vi "Measurement Logic.vi"() -> ()   [LabVIEW 2021, in "Crosstalk_Class D Amplifier.lvlib"]
uses:
  Crosstalk_Class D Amplifier.lvlib
  Measurement Configuration.ctl
  shared/controls/digital audio protocol/data justification.ctl
  shared/controls/digital audio protocol/endianness.ctl
  shared/controls/digital audio protocol/digital edge.ctl
  shared/controls/digital audio protocol/logic level.ctl
  shared/controls/output mode.ctl
  shared/controls/lowpass filter.ctl
  shared/controls/highpass filter.ctl
  Measurement Results.ctl
  <vilib>/MeasurementLink/MeasurementLink Measurement Server/Classes/MeasurementContext/MeasurementContext.lvclass
  <vilib>/PDM Acquisition Toolkit/shared/controls/clock mode.ctl
  <vilib>/PDM Acquisition Toolkit/shared/controls/PCM Frame Sync Control.ctl
  <vilib>/PDM Acquisition Toolkit/shared/controls/Digital Edge.ctl
  <vilib>/PDM Acquisition Toolkit/shared/controls/PCM Data Format Configuration.ctl
  <vilib>/PDM Acquisition Toolkit/shared/controls/PCM Bit Endianness.ctl
  <vilib>/PDM Acquisition Toolkit/shared/controls/PCM Data Justification.ctl
  shared/controls/audio filter settings.ctl
  shared/controls/weighting filter.ctl
  <vilib>/DAQmx/read.llb/DAQmx Read (Analog 1D Wfm NChan NSamp).vi
  <vilib>/addons/_NISVFA/_Shared subVIs/Common/SVL Set dB Reference (N Ch - 1 Ref).vi
  <vilib>/addons/_NISVFA/_Spectrum Processing/SVFA Unit Conversion (Complex) (1 Ch).vi
  <vilib>/addons/_NISVFA/_Shared subVIs/Common/SVL Set dB Reference (1 Ch).vi
  <vilib>/addons/_NISVFA/_Shared subVIs/Common/svc_Log View for Spectrum (1Ch).vi
  <vilib>/addons/_NISVFA/_Spectrum Processing/SVFA Unit Conversion (1 Ch).vi
  <vilib>/addons/_NISVFA/_Shared subVIs/Common/svc_Complex Datatype Defaults.vi
  <vilib>/addons/_NISVFA/_Shared subVIs/Common/SVL Set dB Reference (variant).vi
  <vilib>/addons/_NISVFA/_Shared subVIs/Common/svc_Unwrap Phase.vi
  <vilib>/addons/_NISVFA/_Shared subVIs/Common/svc_Convert Spectrum Array to dB.vi
  <vilib>/addons/_NISVFA/_Shared subVIs/Common/svc_Spectrum Units.vi
  <vilib>/addons/_NISVFA/_Spectrum Processing/subVIs/svfa_Conversion Utility (spectrum info).vi
  <vilib>/addons/_NISVFA/_Shared subVIs/Common/svc_Format Value (DBL).vi
  <vilib>/addons/_NISVFA/_Shared subVIs/Common/svc_Get Weighting Enum and Labels.vi
  <vilib>/addons/_NISVFA/_Shared subVIs/Common/svc_Engineering Units to Unit Label.vi
  <vilib>/addons/_NISVFA/_Shared subVIs/Common/svc_Surround NonAlpha String with Parentheses.vi
  <vilib>/dlg_ctls.llb/Space Constant.vi
  <vilib>/addons/_NISVFA/_Spectrum Processing/subVIs/svfa_Peak to RMS to Peak2Peak.vi
  <vilib>/addons/_NISVFA/_Spectrum Processing/subVIs/svfa_Mag to Mag2.vi
  <vilib>/addons/_NISVFA/_Spectrum Processing/subVIs/svfa_Linear to dB.vi
  <vilib>/addons/_NISVFA/_Spectrum Processing/subVIs/svfa_dBrefA to dBrefB.vi
  <vilib>/addons/_NISVFA/_Spectrum Processing/subVIs/svfa_Spectrum to Spectral Density.vi
  <vilib>/addons/_NISVFA/_Shared subVIs/Common/svc_Unit Label Lexical Class.vi
  <vilib>/addons/_NISVFA/_Shared subVIs/Common/svc_Window Parameters.vi
  <vilib>/PDM Acquisition Toolkit/host/API/Public/Function Generator/Configure Custom Signal (N Ch) - PCM Output Task.vi
  <vilib>/DAQmx/create/channels.llb/DAQmx Create Channel (AI-Voltage-Basic).vi
  <vilib>/DAQmx/configure/timing.llb/DAQmx Timing (Sample Clock).vi
  <vilib>/DAQmx/miscellaneous.llb/DAQmx Fill In Error Info.vi
  <vilib>/Waveform/WDTOps.llb/WDT Get Waveform Subset DBL.vi
  <vilib>/addons/_NISVFA/_Shared subVIs/Common/svc_Caller VI Returned in Error Source.vi
  <vilib>/addons/Sound and Vibration/svt_Single Tone Measurements/SVT Crosstalk (Time).vi
  <vilib>/Analysis/4window.llb/window parameters.vi
  <vilib>/Analysis/4window.llb/Window Properties.vi
  <vilib>/Analysis/4window.llb/Window Properties by Name.vi
  <vilib>/PDM Acquisition Toolkit/shared/PDM Shared.lvlib
  <vilib>/PDM Acquisition Toolkit/host/API/PDM Acquisition Toolkit.lvlib
  <vilib>/addons/Sound and Vibration/svt_Single Tone Measurements/SoundVib_SingleTone.lvlib
panel:
  out "crosstalk":dbl=-96.02835709393884 format="%.2f"
  out "Spectrum":cluster{"x0":dbl, "dx":dbl, "magnitude":dbl[]}[](graph)=[{"x0"=0.0, "dx"=10.00000000139779, "magnitude"=[-102.50662414333134, -98.42652990737129, -104.36739546360309, -114.71774418702175, -130.36950761428557, -151.23179944533624, -152.21861985637932, -146.68742010394863, -149.2705486874169, -158.8294889407479, -160.38776152909975, -149.09872862612403, -145.52257764827635, -146.94377835759036, -151.8503529216404, -149.495187799045, -146.71000188943978, -146.69467169532174, -147.12415322287058, -146.48101024151816, -146.11259440489056, -146.44367304019693, -147.16083048011208, -148.24952674145092, -150.7676188196385, -154.27917637865204, -150.59384849249707, -148.98529072383565, -151.80720194111765, -155.58360918997693, -151.8641272955873, -149.48762329108004, -149.21639953625385, -151.57158440849594, -157.76903119960159, -153.55378069412103, -151.44318082938975, -148.28996695923874, -144.44122146588828, -143.35252367233983, -144.67504951998674, -148.79447192432244, -162.68305251758406, -155.9956623734257, -153.88465520414786, -153.86437747010777, -148.21400992111495, -143.7975301951548, -141.60763781007233, -141.11798493153222, -141.7657625033544, -143.3439946619613, -147.27626397312403, -153.9129306331063, -150.10843385304614, -150.8646772606705, -157.21868893436113, -153.32467973484376, -148.2886012013035, -145.97763528730337, -145.02294775535685, -145.95380075725188, -148.52742611082346, -150.26860428681573, -149.80402808731668, -149.15784362193327, -148.88729473328095, -147.6410694225479, -146.1024386899084, -144.04164734740414, -141.8096017401985, -141.89909839162925, -144.33041994087705, -147.03168187155697, -149.8848916012044, -157.242108057668, -163.7020765469617, -154.84916895378942, -149.35365799485976, -149.84724642155038, -166.16154969079048, -150.02372164994102, -144.4812771299088, -143.00962426465077, -145.06223612725626, -150.044365326583, -145.22102393138212, -143.9047030742633, -147.6498522760554, -148.24512347909143, -144.57573215941838, -144.70421020795382, -149.3992307646427, -157.15858661145447, -149.53376442882706, -145.3500882194989, -130.51626677502895, -115.35893596609503, -104.94632092121802, -98.949745178228, -96.98127597071934, -98.91764337842676, -104.89188220482681, -115.35756716290187, -131.32460144183233, -146.02564661193153, -146.64746502318445, -146.20546432744308, -146.06344187627312, -146.71885957609217, -147.79386540056154, -148.3129984329201, -150.07404032747172, -151.01606867264618, -148.53275640333467, -148.87942637036383, -154.84736140480553, -163.03493024930194, -155.9886526254461, -152.9771504364054, -151.23934598346432, -152.1177287204616, -156.0415527622356, -155.79464630187738, -153.37427864278084, -158.35633010893818, -160.4917326183105, -152.35724216472744, -150.4085235923613, -149.8464780305325, -150.0858277076875, -152.5365543882359, -162.90001265859559, -154.99187315427372, -149.68230609250867, -149.6624222051648, -152.52015170412253, -158.53256622609155, -157.0591968458093, -151.9582556061719, -151.67400414787312, -153.67246366723705, -153.1115685027894, -148.62047969080592, -144.6077065989328, -143.19296640779524, -144.480175755617, -147.26987733162733, -148.8892501068937, -148.0514091905835, -147.536282157801, -148.14352395217057, -147.7677986743226, -146.105745543478, -145.90665814762045, -149.0691401536877, -156.57421189502384, -164.72882020791783, -159.6130972077308, -156.623446560449, -168.85104749052408, -150.1954388285173, -146.74490253016342, -146.42710082184223, -146.06109903695113, -145.11661710541068, -144.87553776047872, -144.76308854188835, -143.36594721535567, -141.29005284167016, -139.77326961768037, -139.65307685067194, -141.68570199128544, -146.42344929092278, -153.22082520634922, -157.77018729369573, -163.00672947759253, -155.66402624536914, -151.72600006433075, -151.90729513417844, -154.055798824148, -153.4554584753518, -149.91810848168632, -146.58444477553613, -144.63227084249445, -143.10913319168768, -142.44048469202568, -144.03441960908424, -150.1025256903153, -170.5464622355483, -160.5458487789234, -148.6474653914609, -142.26330840446758, -140.24130009354744, -141.15484410150341, -144.45679526342136, -151.16119262924147, -151.27648900881798, -142.80993347375116, -138.45182736457332, -137.28603898597132, -139.60807023724797, -145.8636544858835, -151.97115320990244, -151.04114645463892, -150.24123918473293, -149.6371510881664, -150.28927070808865, -150.77161085232433, -149.479675124508, -149.16415541371822, -148.33483632282497, -149.71946210000516, -165.2254495823216, -149.2903130550451, -145.09890222425162, -145.13108280185085, -144.55049294104808, -143.64986368181266, -143.8513304492729, -145.2452116463332, -148.08438161552965, -153.74551065668277, -150.97295897851075, -145.56111974259778, -144.2683578235665, -145.4377665440953, -148.485299942523, -150.606088512832, -149.99901231630875, -153.50105219162285, -157.23107319433217, -152.20302275714664, -155.10568917925568, -182.21878042594437, -155.79850642940846, -149.47657549067756, -146.03673660068378, -144.71418632430388, -144.64436135224898, -145.14852658463394, -146.49628233453257, -150.12506361661227, -159.39136861280997, -162.91970926440146, -163.2211796732435, -167.41114333754035, -159.92861809688566, -156.95423609482174, -150.13886796894343, -146.272968974304, -144.97270598274608, -145.71163317248636, -148.36936121203755, -151.52392886602624, -151.81294816394396, -148.4389448694476, -145.347254503234, -145.0137941154527, -146.21656114414765, -145.71446644721158, -144.26784782916442, -144.8517696110422, -149.3311559719114, -157.19623409642165, -153.14838913323788, -149.80264318689342, -149.51499154993155, -150.0562395375804, -150.46532838788946, -151.81512130027212, -152.08492889376294, -152.27886346828404, -152.96971224616814, -146.00946808785085, -142.63380182350278, -142.67257094910715, -144.48588408268375, -146.4574125986869, -146.8639541246159, -144.39989729111542, -142.6384852492207, -143.3405308391282, -146.01449041545808, -147.77110553826077, -146.78677258658166, -147.80286353597137, -152.5589981112538, -156.17665827599075, -153.973050299784, -154.463102201682, -157.43991958882845, -172.46200114292324, -154.9055892894335, -150.2440233565258, -148.90848142218192, -148.3678538030235, -144.37651973237894, -137.47177539760602, -132.94796185556405, -131.54941025908641, -133.09421788289777, -136.8607463694835, -140.9941498406433, -143.32980767027848, -142.84243382400552, -141.41290900729877, -141.9150734924524, -145.56876843523418, -152.59815574779995, -156.7145964730788, -153.53837597530674, -148.95303591584755, -146.66230348220537, -147.39801912671663, -152.81957024991863, -161.4774498516955, -164.16791044396444, -157.66737544153668, -149.95484667711608, -147.75064574787046, -147.6282926679159, -149.81435262545037, -157.1769895252467, -151.78442822013145, -146.9995200796308, -146.03971538945834, -147.77640124911764, -153.9215633435758, -152.60188744077465, -147.37187720270674, -148.43177928716185, -154.65248382464895, -153.95149291837828, -150.9825556620198, -152.29977978280488, -155.2390354869051, -149.08148104181603, -146.19449053515595, -145.4584987818286, -144.2566970344048, -142.8851826872422, -142.6395736808178, -143.48112329223648, -145.93250198901367, -146.55445027776247, -142.28911808864905, -141.0438316750318, -142.4606533936622, -142.9611355916092, -141.74906552128527, -141.17083672844248, -140.77562836032112, -140.4251709224202, -141.5784061337755, -145.27525608539767, -150.2568137811816, -151.97456113128104, -154.10586925167826, -149.4941602885088, -145.10021934337752, -144.95448872098984, -147.22959951845755, -148.5519093591704, -147.42151523913248, -146.31152370731377, -146.39765371113307, -148.1317610180549, -150.04644464092766, -149.14755515841532, -147.6734828207496, -147.41795159911305, -149.2077277894993, -153.87907767546167, -157.45178914332806, -156.68647377396408, -150.2656499600685, -145.0865782383265, -143.7527692106753, -145.415690876855, -149.4501875710815, -158.52042346703536, -157.8361480689608, -153.4137340474177, -157.30706432079694, -156.4141011095387, -151.83212675449715, -148.7923245236713, -146.32578579596012, -145.4762086973766, -147.26253749848811, -150.45310485787675, -150.6472259696284, -148.4730437307641, -147.85107501340758, -153.67423252222903, -154.10414907771943, -143.32770328199229, -138.0381077328083, -134.4834285265295, -133.5847497838884, -136.2414630969185, -142.09828818205534, -145.92943621139213, -145.24799642531607, -143.78887250522922, -144.08573780081082, -146.43011870617693, -147.15783195784863, -145.92004215266292, -145.68872987445536, -146.164833535183, -146.8753573776017, -147.82392725779468, -149.9187907131617, -155.00485040457747, -174.42491441876496, -155.66154280189093, -148.86628234318596, -145.19322816565062, -143.58136195052955, -144.13634952775777, -146.80034879832203, -149.61413931819257, -148.8639340265086, -146.55103578130888, -146.39749614389314, -149.93126167479267, -150.81086141741253, -146.58075107437048, -143.88919306899965, -142.58041660603087, -142.57992649086592, -143.60532930766522, -146.19675809957423, -152.03286235362984, -151.87476831617087, -148.67005434293947, -146.69500807908705, -144.84575426749163, -144.6292522850046, -146.29427139187112, -149.17942524652585, -152.527120738668, -155.49871242883344, -155.20088215079033, -151.4744693585207, -148.01318050378268, -147.16447927264923, -148.17440278636408, -151.2358775189423, -164.24094842320358, -153.54883070626144, -147.11115687456774, -143.18347079178054, -141.40634376329825, -142.0606833931419, -145.9862099123088, -157.70364335248402, -154.7432383392768, -151.14179490076916, -152.74577633516049, -153.8210209430073, -150.06726015071783, -147.4717662747587, -146.73826403009122, -146.37642992315378, -145.99068626859324, -147.10902970042238, -151.5124661804935, -150.72750323578884, -144.88516599256587, -143.76843749911933, -146.67919575095593, -149.6225698781528, -147.77340235798485, -148.5219342895078, -155.88776205926916, -158.56108756158707, -150.88598313008927, -148.42109292148336, -147.61396360943826, -147.61488159869432, -147.24048439674553, -146.79591949135715, -146.2789993284211, -144.61806349685463, -142.84926998881866, -143.06873771101598, -146.24656998388716, -151.99141888880547, -155.76590877492575, -159.44241264173522, -164.03130545762332, -152.8840073886675, -148.83043565486662, -145.716990740156, -144.2003042331101, -144.33425516969368, -145.10960426567212, -145.9365374278638, -146.81472254195856, -146.4345290735593, -145.2103529379687, -145.36548613378318, -147.51305715920563, -151.28945507478844, -151.083216869563, -149.18053233854613, -148.09222412733868, -145.32141880018193, -144.77249531781612, -147.08648253059596, -150.57012243898464, -152.31341238411954, -152.30808120657758, -151.51140561026506, -150.19385147721778, -148.80615432403738, -147.38603202824723, -146.85926929339576, -148.35043741286563, -151.90878138886697, -153.72930692938286, -155.00835850985632, -154.06879749319023, -150.35094978081676, -149.69253944652456, -149.9252932477334, -148.38310709651697, -150.37799609657742, -154.01091995660005, -150.09939439617452, -147.0463412503836, -145.59619446670976, -145.69144921786406, -146.90009115209813, -147.9606174292869, -150.45381822586697, -160.56360004338967, -151.10238463377092, -145.88882121638156, -143.6838315166682, -143.38823034066382, -146.043971263991, -152.38791210229562, -161.28227008781747, -163.31420065793304, -153.6149198581791, -150.93150024864195, -147.0190093538344, -143.37490209684086, -143.16078098340452, -147.02019254694116, -160.84112995140185, -150.13875109997124, -144.50392468710555, -143.3410847032433, -146.5290473219592, -159.33783477619238, -151.1705556837585, -147.6092302048642, -148.12543112524972, -152.52113246534793, -158.09159445791508, -149.33748162636942, -146.80594890391419, -147.59093397079175, -151.47331855354363, -153.73865203546876, -148.4227558103694, -147.02007200455193, -149.01240505083732, -149.93794025206648, -148.49559024766896, -148.32345675886904, -149.47271093008303, -151.64927194659552, -155.04241373726674, -154.93021175148095, -151.3593771769159, -149.5302414147572, -149.58099385197, -151.35888733398903, -152.655194503017, -151.21584226486635, -147.71016819107712, -144.53661775483846, -142.80741553660886, -142.03359293145385, -142.04702604631055, -143.2096810280472, -144.62659937726147, -144.66747259756676, -144.4882336612964, -145.25491193335785, -146.87565476403287, -146.68515285444192, -146.0797944282166, -147.82589874847713, -152.70476511685195, -168.87729485966872, -155.07308060387894, -151.75472336609755, -153.5078432751017, -159.12452243970995, -150.28532558393277, -145.30950410750464, -144.23369879322823, -145.77244639789413, -149.24410947939407, -153.33791001921026, -154.2873685466283, -152.74781696520603, -151.34834675502813, -152.01259026184331, -153.57977168578833, -157.89033262422848, -167.8209490947487, -158.69160512614386, -152.218824584785, -149.7045903062854, -144.94862049864142, -141.92812754149568, -142.11776317394754, -145.47281721849546, -153.70777689164467, -163.72689103274215, -156.5643861544259, -155.0095207475167, -147.7379997485942, -143.47701616544725, -143.66431802411174, -149.56299569828101, -163.18788928712067, -152.33262143279748, -149.70761324335794, -148.3557160900782, -150.1285207782886, -160.81898385526665, -149.30172832474233, -145.1415394648689, -144.55889071528725, -144.60228698556645, -144.89492976864648, -146.01929483160416, -148.24639101703238, -150.7118047226229, -151.36547068783545, -150.28922326303197, -148.32875603939303, -145.4847902263635, -143.08833194205093, -141.79590189361483, -142.78125897673422, -148.65567654490422, -152.34289308858297, -144.58987116399894, -143.5193242462612, -147.42445073377738, -161.5001866687884, -151.90577900704707, -151.78801441605484, -150.6843624341204, -147.5706096308335, -147.84464876440956, -150.0441490627542, -150.26055266489732, -153.6837029294246, -159.85756154833234, -151.03548535977387, -149.51755087584283, -148.8797238211103, -148.38149518659182, -146.38226649290712, -143.92996587846494, -143.62278734456567, -146.14810714577428, -150.24880344759748, -153.7751642391114, -166.35323726065576, -157.68643617441697, -152.20397418932362, -150.9255092415771, -150.82539938766595, -151.6381635151032, -152.360545981892, -147.6051161178156, -145.32201535304472, -147.62731708257922, -153.77136850606172, -151.87354306901534, -151.53546848432364, -155.6549499973205, -155.31442449960747, -151.79015844191042, -148.6165583275531, -150.2025924180614, -164.7944423463329, -150.70632065394128, -147.10040132520592, -147.6991730897426, -147.7472703137542, -145.70859612333552, -144.1234458919444, -143.3965255845766, -143.52019473030867, -145.35246672227046, -147.15677533212266, -146.3067841440703, -146.18882730406784, -149.19840869327547, -150.69008212777564, -152.7887806504483, -159.43863294580933, -145.62078604901868, -141.707054723239, -141.63690262044435, -144.4032915477667, -149.51151594735973, -153.24698568235024, -151.41471562308712, -149.3113746303565, -147.7508328212677, -146.72205766212866, -147.27502901759198, -149.3806654540449, -149.46961992297514, -149.0293079638374, -150.36123728176693, -153.27926501599632, -157.3798113515253, -157.8377747386401, -154.7515489375611, -153.55801345507413, -153.1134030816651, -151.44823229899308, -149.39572935811913, -146.74405428109233, -145.79827537476876, -147.92175748915017, -153.92428321974836, -171.1409828123313, -154.87077152335982, -154.46593567427217, -155.8753712851411, -151.74062149076923, -152.88610210753484, -168.64643295262647, -149.59109525891597, -145.62075790485994, -145.30276996356545, -145.4998321569811, -144.36887727675764, -143.3554362478537, -142.46708259933803, -141.03535447462892, -139.77869805413405, -140.07103781652313, -142.9252859267721, -145.3429096708324, -142.75576019099387, -142.46837445843906, -144.8093615481277, -145.0036215989304, -143.655315246657, -144.76417998665397, -148.70919245082666, -155.17236700917832, -162.78754538681022, -159.6303106965218, -154.04408077705935, -153.9081005762546, -157.77442088159867, -163.88536985065707, -159.18529597020495, -155.7260851578025, -154.4021989532899, -152.16312876807112, -151.70950634629315, -151.37930402590536, -149.10065090260244, -148.55426443806914, -149.01150370967045, -146.34022717878327, -145.13002220149994, -147.41043607311337, -150.55698219147476, -146.60316480686976, -144.59851104600003, -144.52424108187816, -144.11437192001603, -143.28135154567116, -143.7973673988034, -146.94343771609928, -152.16981315262564, -159.4509162420397, -160.6977127581841, -151.9199036406186, -151.18343341106356, -150.38936002427195, -149.47195927469073, -151.2645280861349, -149.69005604455484, -148.4060452573165, -152.8933723640657, -164.17349635373643, -160.08845562476498, -164.10384305316302, -156.20955896824978, -156.84490253915655, -158.19345624863746, -154.30245511754828, -148.90559869008734, -146.61618381923174, -147.8055603512899, -151.1262101560643, -152.5815846908356, -153.67023258987413, -153.12928967194415, -150.15865778635114, -148.24441170472033, -147.8174846326163, -146.2784837811589, -142.83503841232448, -140.1257089151161, -139.79683568775008, -142.00605201575397, -146.24173893325315, -151.8208600706655, -156.7231115740033, -157.28590560542014, -163.3605332745614, -154.28788064592015, -146.76328569990622, -144.91571346538402, -147.24985043489696, -153.51189256971267, -162.8894889720429, -167.05408999060293, -164.48260306424157, -162.94455846657348, -163.11389007382743, -161.9745045209098, -160.78884210639256, -161.3300961569645, -157.56411248378242, -151.42835835673407, -148.0780166825534, -147.40898172690015, -150.5461189462095, -162.93817400865538, -159.47686703014693, -162.6906488635256, -162.09386589690652, -160.87487880592417, -159.1170776844069, -153.7423208183152, -149.90202111555948, -146.6887141029134, -144.1605112970981, -143.0126790654884, -143.84900527797964, -145.97484503322298, -147.57480777439017, -150.73127106168386, -149.69212111284054, -147.26828787740607, -148.30082792971584, -148.35921452475262, -148.09727117793665, -149.27025579146135, -149.09668237619198, -147.22438950463297, -146.0274369547106, -146.14558039698906, -147.57029885604157, -149.6419510688468, -146.14535671921462, -143.77803691261948, -144.53821790207212, -145.2899709943745, -144.88594248662696, -146.19345056466523, -150.4170528087398, -154.41242797733915, -149.11787829209175, -146.91262431204694, -148.32709965534303, -152.61889234068374, -155.83639579471873, -155.37391741265264, -153.59432967747085, -154.55906085111693, -156.35911529535818, -152.09412507360167, -148.17032431704897, -146.1254638444616, -145.12794497600993, -144.29752212116034, -143.84795320248134, -145.0894181085908, -149.0188658920894, -152.241962094018, -150.16180212463104, -151.10592842944504, -173.9609656213844, -148.03805539242938, -142.30276044684115, -140.3881543820158, -141.00281444021735, -143.9970311902058, -149.00329609206125, -148.5559736889403, -148.1288390037594, -157.55397577790052, -151.6941905670164, -145.87818248212653, -146.91829112658644, -157.63119764767552, -152.52544778742455, -146.9718405834502, -147.24188450325295, -151.43372095109785, -157.70593114313436, -152.15159975949092, -146.74926479872676, -145.2279775722699, -148.7542448291814, -162.735809358672, -159.70394271345253, -160.5390329988378, -153.91546744769335, -151.00412933429655, -150.2637120905425, -150.24691085398754, -147.37930282659048, -146.95652939924054, -150.11013737003515, -156.61909308462555, -155.20053031987985, -148.72035553942507, -146.3317228795784, -146.6543971154827, -149.0761943243432, -153.42357549817712, -163.09680022715816, -155.08208146674548, -151.79839018589504, -152.97133209381244, -157.1811911561128, -164.7556538517111, -166.06385697443318, -154.9499476656444, -148.8910148015049, -147.95429545674597, -149.9573485232521, -150.10081059413227, -148.58819100792851, -148.04592263520857, -148.11519918770782, -148.91802354480933, -151.30771166709619, -157.2183335689563, -161.03866717485397, -153.64654903299441, -153.54458668066673, -160.02418141724948, -153.191236215802, -149.33725849472714, -150.52250810728455, -156.95609661275475, -156.5638612113236, -151.52878495970606, -151.1781240892623, -155.53457880339064, -159.89134443673447, -151.6729535054317, -149.5683500848053, -151.46948234777054, -149.79043276728467, -144.64566630556394, -142.29440847841624, -142.40465212808823, -144.91679336045794, -150.84887715570736, -163.89194329804238, -159.6976039252596, -159.31332729018163, -157.3422842401208, -154.72447123098954, -152.90120689788435, -149.03862097364248, -148.50013894376906, -149.87206064582574, -151.70055177773298, -161.1728003584105, -151.79491088552055, -146.4156376315854, -144.0342243751101, -143.5184349766976, -144.79611130968675, -147.54595298722305, -151.25435024294723, -154.32553778520077, -155.80240079088594, -155.9617921500691, -156.2318885349061, -147.24182046912577, -143.20467671320267, -142.8016619489143, -144.3624492748015, -146.2398728953396, -148.18728807357496, -150.4965035250082, -150.35016796748056, -146.4870423315109, -143.24522100555743, -142.48076093913008, -143.90492503994085, -146.29794201729868, -148.0743010389357, -149.86678390384088, -154.9477907282562, -186.33976288851247, -157.1081505983334, -151.1254128321099, -148.98918927409494, -150.53467850208798, -149.78377847630938, -146.3920650026197, -146.87035712787218, -151.2592817587066, -151.7571519205439, -147.636024541987, -145.05498201867863, -144.4542620933105, -145.6081569983016, -148.76005468423836, -153.87384117524013, -148.98306402573044, -144.23604419378424, -141.91831309888866, -141.2480330231254, -142.08076206252937, -145.0927810170704, -151.14221046205344, -155.73475478904788, -152.9086049103152, -151.605493665403, -152.1771745251403, -154.52844596344562, -153.6828464169662, -152.4593113724324, -155.7524731445178, -154.5702346277548, -153.9710825666257, -154.74303627785977, -152.5364274376303, -156.14988305170596, -156.20335505615407, -150.26400265338413, -150.45903506924412, -153.18710436707113, -151.07908221037673, -146.85630845551407, -144.7264667924648, -145.57680928683124, -146.4830265191285, -145.28614435758976, -144.89467099680115, -145.72105059876233, -148.53526568722438, -156.11524456827428, -158.12000842811443, -149.7536690985783, -147.05367506488452, -147.5675271519732, -149.7679862226397, -148.56966478820027, -147.86339166213986, -150.12480554677518, -153.21758336607655, -152.0790532051706, -150.91666761931754, -148.14843365268925, -147.00885672246753, -149.06073046689065, -153.8331332376428, -161.49885580784104, -155.33099707813193, -155.6904047087652, -159.9797634299892, -154.92380658865517, -149.59368982016179, -150.35717608423226, -155.5389166385462, -147.59696110320397, -144.091901827543, -142.52430502578096, -142.70414951722543, -145.27089332353324, -149.30600171138974, -152.01710569509308, -154.26508114051362, -155.51139016303478, -150.74859132379262, -150.17570465437598, -155.49388574234214, -155.1516219536232, -150.9261526297986, -148.16472748321854, -148.3283456324221, -153.32212121554215, -180.24244029664868, -157.07471738613572, -155.8993576189565, -159.5595151877714, -159.80387813697334, -158.06772482772965, -152.15457329618343, -153.18595201271387, -152.92717209950945, -148.32412453286622, -150.92734734223794, -153.58741924500686, -146.03905914852572, -143.55198411642073, -143.8834611255214, -145.80421045496718, -147.89706608341146, -149.73137302485097, -152.3156858002491, -153.48165871092814, -150.61028370340347, -148.79223306865597, -152.03479075687787, -173.5299356817588, -158.68858939957428, -156.26938003914472, -152.48622691462617, -152.88256503885194, -165.19729955689456, -151.62818965820128, -146.58984601313313, -146.60296677858395, -152.38659607411498, -157.22837512519243, -146.83611440283428, -144.73791399321988, -145.89347884064142, -148.46048074181525, -149.2672750648801, -149.27034882684188, -151.5825298754759, -155.37954908264166, -158.85908048131046, -151.80154831474985, -146.30540344607678, -143.7706433816793, -143.64153842290352, -146.8370197879104, -152.81335451353652, -153.34318511506143, -148.01616977503784, -144.83575212854282, -144.7672564885568, -148.3385021436814, -153.8372732851474, -151.8657690860778, -151.82556494243136, -152.3358521106764, -151.1016350783282, -153.92830553836654, -167.43874507608012, -159.45613395748174, -158.8803353575257, -161.56426476439987, -160.3103934790014, -154.7735128499723, -150.9703191982086, -149.9165416725486, -149.08651994462736, -147.88516851607514, -147.53345714364815, -148.59160245065627, -150.44350397635876, -149.81085432693453, -146.10201804754948, -144.8371294767596, -146.86442700852166, -155.15102407883467, -153.79624802580543, -147.23057954978725, -146.73797967361736, -149.4753545898011, -155.90516562744213, -155.82963084709573, -147.35437352818732, -145.88398572616654, -148.6103808468148, -154.3718071675014, -158.9547618139327, -159.19681555936648, -155.54190967813543, -153.09597522450935, -151.11612137563947, -149.84675931203694, -146.83124223360917, -144.5239704315825, -144.23068720734892, -144.69702847742053, -144.2350026835172, -143.66742252197315, -145.00745530730072, -150.80278915702172, -155.020168071857, -146.9802909607082, -145.09156057395106, -145.35995538018287, -145.80497150907863, -145.85885836721107, -145.37576795087244, -145.72655094767757, -147.8221980877563, -147.93487472473646, -146.62902180712967, -148.1510107221433, -153.99667340505596, -153.18875540920612, -150.53237940442193, -151.44737105738474, -147.61859489543195, -143.69264150874676, -142.14950731866298, -142.29581358315988, -143.8765815127819, -146.86792107615813, -149.4551646256768, -151.97907410845866, -158.54114270158973, -169.22096369559412, -163.25234006832457, -156.99812379258216, -149.44132815044995, -146.0162553540373, -145.61988509776262, -145.72293391945385, -144.89134400923544, -143.44564874151726, -141.94704039462033, -141.76375984240772, -143.78382729882043, -147.81345957210485, -148.60834263464992, -147.98686809393624, -151.49620929713248, -152.02106339217397, -147.16207558023052, -146.27063713331054, -148.3563441924551, -151.6142724116232, -153.53269515847154, -148.86389839522963, -147.7393001826794, -152.1840346886108, -177.93110433743573, -155.8803796690748, -155.09045562105695, -158.4829101653637, -156.28434298223232, -150.85676043464034, -146.18980549571836, -144.7453221983244, -146.93355174984146, -148.82579983582144, -146.2638867074142, -145.57767540693175, -145.01639156108521, -143.74987650286508, -144.83723639098707, -147.06623265441627, -146.05145486511313, -145.33125227207674, -146.59066050255743, -147.2872511435517, -147.30819204800568, -149.14796793727038, -153.2380237857195, -157.50095131028536, -160.88540430939102, -154.07941114477916, -148.2635919891576, -144.58408777109446, -143.4403523940984, -144.7931392139378, -149.23205322624193, -160.81279199620815, -145.67252152028678, -141.04820858350672, -140.32487525433652, -142.4465482222109, -145.82996815275575, -147.46952604101043, -147.82483183221922, -150.37007176830647, -155.8814528554197, -148.43711642945016, -145.8656072238287, -148.84186914694794, -152.50591139270557, -150.32065141376256, -152.83281580901925, -157.20707635417432, -149.11176768240654, -145.00810537121419, -143.61545115883206, -144.10015940989285, -146.95427726954398, -155.43690814041616, -158.87346763294028, -151.39827820991923, -151.00584645861977, -151.04263698210866, -148.57023870920958, -146.32422713761773, -146.59584761301625, -149.5316785774225, -152.52083151358147, -151.58657864670104, -149.1872678830132, -147.12986521271483, -146.2571337818404, -147.1816935549501, -149.70967843446786, -150.27944610411834, -147.65714391108793, -146.69068151990854, -148.30113399435322, -149.47242224638111, -147.86143704503976, -146.79616260915748, -147.2675252430356, -149.0583272568076, -151.37529287129195, -152.15255617233146, -150.9230249236825, -148.90388378377583, -146.72768465791418, -145.64330211282635, -147.2113530957228, -150.72813591137356, -150.02426537389567, -145.6463318226989, -143.54438874460777, -144.37347054544267, -147.48945725596369, -150.7159222687941, -151.25225081865577, -149.89983616876293, -148.15657981021585, -145.65729141552356, -143.8101294024512, -145.14713782138134, -150.93706553025928, -150.3160957879936, -149.8093998478747, -156.6687183510309, -148.523091987029, -143.99629233733705, -144.18546136811955, -147.99317533455334, -151.4290192616181, -147.89512329646615, -147.59164191611484, -150.59622572664043, -153.87350523752505, -159.49907680473896, -169.48560572374544, -163.60650809898897, -156.58936131632265, -149.85021438952725, -150.03514073683948, -149.47510312877895, -149.62021615638295, -152.89600528521035, -159.70937348418846, -165.07005018218655, -151.95942512114786, -148.04101382852025, -148.61343204823427, -152.34562474604053, -151.81207663100486, -147.91744874116432, -145.30103395765192, -144.1355464386679, -145.05060017414021, -148.09057761675408, -151.41849553993634, -159.61308082382078, -155.1816523646556, -150.5913322256098, -153.331116541228, -158.52751767432105, -148.23969761346677, -145.5526272186985, -145.52872877019962, -146.23637423102093, -147.36639252286525, -148.12241917826316, -147.22456989388706, -146.2634886877461, -146.52306251159655, -148.70522791045633, -153.4382669938375, -155.37305449870794, -155.11555977393047, -157.41855365755652, -160.71090544479733, -161.09680006655708, -158.5936830027534, -158.6685162996653, -151.1749230904655, -145.65934281971212, -144.43461830432193, -146.34988189325176, -148.7638477380629, -148.01229742201386, -146.77587944765523, -148.2992511254092, -151.9986978497002, -152.02016858590162, -151.7298260325462, -152.4925386930184, -151.9963983649795, -150.55779112097187, -151.2679219601771, -150.94288128269073, -149.70741870665452, -153.28217184138745, -165.55276866709093, -159.0851312068457, -166.85331075535424, -160.44539250728545, -156.39808209799037, -161.43984025334368, -153.22710376789098, -149.4256909851157, -150.18838767732308, -152.40658915448148, -151.76186957140612, -149.96158574546595, -148.60148953879397, -147.84484383577814, -148.92610623543808, -150.84415770519243, -150.5877737248299, -150.6550389772269, -149.80873786753494, -149.03218189108713, -149.9336211366658, -153.4096127113656, -154.80965967516903, -149.76753112422904, -150.80253440411875, -160.60073329888633, -159.95514758555893, -164.276491905606, -162.6227968860655, -154.53462235325952, -151.7646022947383, -149.5887047318782, -146.6785795885124, -145.3583898893711, -145.7325392161106, -146.61998224994372, -148.69088006998672, -155.25513837198534, -156.36538004922033, -151.0103529408843, -151.0952581617615, -153.70573552360224, -158.85278043347208, -150.35390545516665, -146.09817943558534, -145.5542681042812, -145.1071104691135, -144.15009403852864, -145.07490966040265, -147.3548713261334, -148.9506283802712, -149.68608795724438, -149.65120343477363, -149.62071988097, -151.1706352141977, -154.49867904845703, -161.36928869657277, -166.2725270601443, -153.97163723541433, -148.65175435624474, -146.5544028635628, -147.07115111037677, -147.92888140142108, -147.8639066626015, -148.4753248006793, -148.81166037890569, -146.90427077360755, -145.5407368066807, -145.06999849045053, -144.29699872257387, -143.67545179821857, -144.26500529883074, -144.889370647509, -144.7156812690359, -146.6114980199243, -154.3723109288688, -156.2623007976317, -156.43467614096875, -163.08770361193538, -157.73096871036896, -154.83265189265944, -151.18182308131858, -150.02823798332398, -153.74371212280695, -157.7986664563576, -153.40276620001097, -151.10284689614954, -153.13690532712283, -163.40254085963096, -153.4265176720444, -150.44170958436072, -151.63297520885493, -154.53604009593874, -158.56784314141555, -163.8619563753645, -156.19829253949723, -156.38055327417842, -162.90270374384247, -158.57150148069672, -155.42328957198333, -157.27583115741785, -164.1684582892087, -162.16160283193472, -150.4172778208516, -145.72850283694805, -144.98853856667606, -146.35754904330318, -147.4929200056926, -148.2949411628738, -150.9378325510731, -159.39621014125836, -162.23909398076268, -154.33512182189395, -153.46038747401184, -151.79073260120023, -151.26638526988364, -156.37121704211614, -158.54789930914797, -155.1952497580852, -156.2233090939976, -156.00344409609596, -152.63809916480443, -150.42340297694253, -149.62109747104964, -149.97567851673898, -151.74730935398793, -149.4951066741491, -147.5944363978778, -147.26796971646002, -146.80683518631298, -147.17544408214422, -149.42248335742644, -152.23437753852704, -159.06757296744706, -161.48825055747355, -156.0841706168236, -156.5304407109267, -159.34541572030116, -158.58572962316038, -151.75968423385723, -148.02471324972052, -146.04989691536485, -146.2198396634561, -149.78077705587313, -161.06906213008688, -154.76411440797773, -150.31425672601335, -152.03080067857582, -163.6143142711507, -156.61855099884434, -149.3889789907917, -145.96086390554157, -144.97341134116064, -146.2109021232264, -148.48074566253308, -150.24644567835668, -151.34118045723784, -150.49908090871708, -148.31592415868943, -147.05912185430842, -147.97971259907794, -148.85996943853814, -148.24285129254267, -148.47591216151227, -149.99398021302366, -154.60877553301367, -160.78227655894423, -149.13810338680514, -146.67610087943328, -148.54931540246727, -154.40698868959967, -164.8581254123114, -164.7766463890734, -164.47815425349103, -158.82619729601913, -150.51169906623042, -146.1263901636695, -144.33821891983493, -143.63157207562745, -143.31220520097486, -143.31109195571028, -143.74330041815563, -145.2513931321165, -148.61560509864032, -148.40365227861446, -145.02150065312156, -144.10462071733446, -144.57586837370312, -145.18843763341636, -146.21992657641607, -148.93984205396345, -154.71078519420433, -162.01652636118462, -157.10995984924313, -152.01425475532724, -151.18942560792084, -154.5984107428198, -159.88851916308414, -158.1478469050088, -154.5499387406346, -151.40362307414935, -150.90680635010847, -162.25474391188598, -149.91528233144297, -143.9060843432841, -143.57494667735503, -147.54924537580823, -159.32408709059033, -161.62539421183365, -161.7087089291656, -167.48263956657948, -155.61108335750643, -150.60060683588082, -151.20289995693935, -156.02223983684388, -161.9223110810243, -161.31301297295897, -148.79202349251642, -144.55854953640042, -144.28647107050585, -146.95872016072147, -148.73227778926028, -144.6927470839806, -142.77434497707168, -144.47735139793303, -149.7644357894964, -149.39894547567047, -147.1162105668714, -148.65316695552085, -152.10492406885086, -152.01367318354795, -154.12357117465223, -164.16756599200755, -152.11413657871995, -149.20701565457603, -149.03216356399122, -148.93056469781655, -149.33463153954858, -150.21348361876576, -152.1051536220831, -153.42475161632075, -148.95322401521125, -146.65815723244702, -148.7335155111253, -155.82828383314674, -157.4901579827059, -159.89952573365957, -167.94483703333668, -153.07311813479086, -148.35121909906175, -147.21723585006382, -148.21588203753058, -148.7984010712621, -147.90973915223003, -146.5033105109343, -149.20048961887107, -164.2240893640785, -159.06746477529398, -165.03039480500684, -158.61273940182184, -161.4035143297173, -157.87308382656082, -152.11667820329305, -149.31347990256134, -145.67653143812953, -143.78855058763168, -144.96155957581468, -148.78532087601033, -153.8134466289772, -157.69407551809093, -156.5002888919415, -152.9574810517872, -151.5639216933444, -151.46830533106868, -151.1866806019993, -149.28638525164158, -147.68905556307047, -147.0961368925848, -146.818075718628, -148.8188549013776, -153.6062583707522, -149.85304139134206, -147.08808447543265, -145.92588195635375, -145.03628951176222, -144.6337687359954, -143.66046908772103, -143.5089755443044, -145.38982791629147, -146.55549866493965, -145.04826569947497, -144.0310569895553, -145.60500316540822, -150.9261785240022, -154.46709551738033, -148.82117093891492, -147.32711757342375, -148.16037487707436, -148.53129811331132, -148.05179889439805, -149.3334386200684, -151.5183497722668, -149.0037406263837, -147.07888095895106, -146.38265885153493, -145.8967431800232, -147.25105060396098, -148.64527193577413, -145.707381255305, -144.88613423000766, -145.88139982385567, -147.40027337935493, -150.5658451746915, -154.294130565827, -153.1822008626875, -151.09919755631554, -146.9259661838833, -145.16033044566572, -146.59423008337143, -149.0847385500971, -148.62634594475273, -145.93051756210292, -144.66252298920534, -145.75298080131358, -150.2478031595255, -170.0197436153287, -147.3754623787009, -143.4469873354932, -144.17590566231112, -148.66877588192406, -152.34974981067555, -148.40394120630742, -147.09896007517506, -148.46926464561517, -150.5312526341218, -151.46451270393808, -151.39338121347163, -152.0464175899192, -156.3513202571602, -156.90570998416086, -156.94711267745697, -163.48408780043317, -149.8482737249898, -147.03621728576903, -148.9091532548067, -150.36811217738972, -150.46537476067607, -153.16265632200378, -157.22236918864556, -154.33733505957906, -149.86741949150104, -148.35369337490616, -149.1387285010467, -153.96384032124968, -154.54608126640963, -150.1259605317498, -151.52059991166402, -154.91862673508118, -152.8317807257511, -148.74388724379241, -147.9556219924176, -148.83638352710025, -148.16398020560615, -148.81054432445146, -153.2951941482244, -161.29352038167883, -155.52313944693861, -158.0146098796669, -161.72492184478222, -151.09287341679953, -150.1525043171416, -151.79731815694043, -150.39503927072894, -147.8270383710625, -146.54585873813846, -148.0367328579057, -154.44532691082196, -172.9607776422613, -165.27157542386746, -162.73906005949814, -152.37317183370703, -149.42652383346172, -151.73626601595996, -161.00229716670975, -151.99195604819917, -150.71699570431355, -149.62782263354927, -150.63443109143836, -151.687559658298, -148.3100415986531, -146.08810383074686, -147.50212604085985, -153.88197749107493, -147.067072012468, -142.3613013728353, -141.40249151096077, -142.04151726318605, -143.29507935118426, -145.2515561713242, -145.57048291801533, -144.67014646121993, -146.59841990965728, -154.56966769201438, -157.69331188245388, -152.5830223698453, -147.8792717976901, -144.6069964420152, -144.53635992666793, -146.01627398518252, -145.33680342213304, -143.85344607473394, -143.81753685591315, -145.60152486207534, -149.36382993534176, -154.98582426741604, -163.1188282214397, -165.3808245913842, -161.12020470301252, -163.24230061005065, -150.13871035884847, -143.48671575709406, -140.77537020254138, -141.27256092057078, -145.24407314544283, -152.7394176585167, -157.10848628668168, -153.94443682179642, -149.66364686335749, -148.39327124041782, -148.4803233585021, -148.64614889621586, -148.4354732796072, -147.51185590276216, -147.2102819265351, -148.69383445064796, -149.1166954089549, -148.35870329054598, -151.63353252713645, -168.98903986070496, -151.374229504347, -150.00460295354725, -154.2350882245497, -156.18430513078272, -152.82010925843082, -153.72876016452017, -155.4542038762, -149.7320363566708, -145.90050774452033, -145.45130463892914, -148.05549763888487, -154.13559555247815, -164.10327472943771, -158.6588822737728, -154.18905532402508, -154.17931385054746, -158.95426452350185, -161.26657260612077, -157.12793549969783, -150.54359304795813, -146.70114855809243, -146.36621565882393, -149.48899825382307, -152.99742263832397, -154.93424722170258, -161.55068836259457, -163.58271782581886, -152.82878987463678, -149.20648120735598, -151.55739896891856, -150.96618317530363, -145.7529642969318, -145.13803760407586, -146.80661654923975, -147.51697106988377, -147.71474162254253, -149.75562005895094, -149.58894440705296, -145.7788355626545, -143.90014220645543, -144.12159276760786, -144.47287699201723, -143.76829652460356, -143.76740402743087, -145.81017257783432, -149.0381973383115, -149.7460986986614, -149.59442311440108, -151.0759739869577, -151.9563662478458, -149.31870796651597, -146.85842291803516, -146.48582126711366, -146.8601782775804, -146.82726297521054, -147.97717717424692, -150.3702318653182, -152.1300178941021, -158.68198703810003, -153.60870176936731, -146.02961105679884, -143.39445126296033, -144.25332961125906, -150.57615596686514, -155.7532185012074, -148.76486923917506, -144.79843397139396, -141.78595043420515, -141.6953128513235, -145.04390285825377, -151.72337576640405, -156.2845162443405, -154.76975655835395, -151.63299415703062, -148.65368249780005, -147.12731020623235, -146.47832280752414, -146.36699725670496, -146.85049803323753, -148.76959427598058, -151.170595422532, -149.86483149552737, -147.2659220926924, -145.41513257456347, -143.96558702586367, -144.15773000265966, -148.69766875542135, -155.86232996961328, -145.34463498340466, -143.15658169547555, -145.65187989130538, -154.48897380892927, -169.19823774944857, -166.99191748586264, -154.39243550539558, -150.71171416709032, -150.31868961063395, -153.42630253890053, -153.52974881392905, -147.37163434916943, -144.907550344246, -144.87469329676804, -146.7969394365554, -148.6929987763437, -147.5840529418228, -148.14341123024352, -149.32494701732824, -149.63785684310574, -152.33075908617928, -156.3824461006963, -148.68568271920986, -146.99783002027493, -151.06116343556505, -147.44299463931677, -142.50887829004432, -141.37745894950032, -143.30452093747374, -148.52996698290298, -155.8855838322915, -152.9225748698881, -147.69733459939175, -147.4204922572643, -151.26013003927878, -150.25712407557717, -147.72190344008004, -146.05136044953485, -145.2276597064361, -144.20747817340722, -142.94891831986922, -142.43763693302526, -142.8694340616852, -144.35133204271193, -147.51740968504132, -153.29016058346315, -154.46932241555814, -150.99852551621214, -152.82783852273272, -154.52796139468177, -147.2225900262727, -146.62318318523538, -153.64068635281913, -148.4600732979263, -142.4263608302064, -140.12411659916538, -139.49121156075387, -140.1661943644832, -142.0502426024817, -144.2706020145182, -145.8340693065945, -146.8433574370072, -147.2120657695626, -147.6189722306987, -148.02875363514084, -146.8298982294483, -144.08757447116565, -141.89203243370517, -141.84264066796658, -143.49044470264448, -144.81061200821262, -144.9245889058699, -146.92359730062807, -151.8975183901755, -147.04811307860794, -144.1621244649547, -144.42553226715614, -145.3220388997423, -146.00433333882447, -147.1852217953072, -145.97025256823665, -144.08403866671992, -145.02182688514404, -149.50478525863312, -159.29982960116482, -161.4954577988094, -164.51915819942712, -158.13521490257037, -150.9601717890434, -146.75761354951393, -143.5329816906841, -141.91672565676515, -142.51176386694542, -146.73245664611233, -161.2880102074384, -147.65533826725888, -144.08431454737993, -143.63456076812935, -142.8385084622302, -141.58443858843367, -142.28818712308893, -146.33942093561382, -148.3883647228296, -145.8856124256247, -145.86627026866194, -146.682367231984, -150.23631026639524, -167.04190338935572, -149.8604206950048, -147.90238217006583, -150.5873061371969, -149.62462870475787, -146.91444989234844, -145.86620123964525, -146.45226160352553, -147.7631359082479, -147.25746863677048, -146.18111225700937, -146.6075830912884, -149.13658205306325, -152.55716024938266, -150.3533066242655, -145.90279541275595, -144.72430459972847, -148.00879112981255, -155.42642713116874, -149.761968872363, -148.26044637371234, -149.35781027407035, -149.9784227580281, -149.7897266690288, -151.50048670300916, -151.48818208957397, -148.01058049770938, -150.17027965938072, -167.4063988389981, -148.37825113823516, -145.6167709142772, -146.7932609048282, -145.12660230473958, -142.55766423794344, -142.8325805415466, -144.5066925134135, -146.9281674903774, -150.18903700645484, -149.67990455251743, -149.3288463329665, -149.3113081322508, -146.44359846422245, -143.67964196567, -142.04284979458066, -141.2885975981226, -141.46553301540646, -142.50360085266095, -145.86845897018648, -154.26552979719506, -161.08400968120523, -153.73319723065276, -152.06080945505386, -153.91922732184267, -176.6511136331209, -150.81334834413843, -144.83196502864084, -142.9638702734907, -143.52742385566563, -145.4244401774779, -145.52945709209484, -145.30457556507517, -148.72735521988272, -159.374839920016, -158.6917493479805, -152.43275515700557, -149.3737511408113, -147.95094825386604, -147.48392785132586, -147.67874267410411, -148.82510619766234, -151.36938231894055, -157.02164538839352, -159.12463166961106, -159.40234773685953, -160.87923709093565, -149.51730009562337, -146.58133295182492, -146.34086080239575, -147.5626612041442, -148.9209868352458, -146.1813035561077, -144.0475373461267, -145.7409563237111, -152.32909241222177, -164.73847750253287, -159.31835313271594, -153.43746356910881, -148.78638606849532, -145.79304343500274, -144.41712140146865, -144.02673116802526, -143.85898100702025, -144.0907450753127, -146.26795198025513, -151.2207241639404, -155.16243729446242, -157.63828914045231, -150.3521379158742, -149.0949640747826, -149.1585700673466, -148.325569939181, -150.9337149024033, -158.91354118680894, -159.61308287740005, -152.0272684839231, -149.12717091537334, -148.60307422727703, -147.25779958568165, -146.55164682938383, -148.03840565485228, -149.94397048233355, -149.48812213873003, -147.45304591835503, -146.48021746840953, -147.8731246925875, -152.2034763307141, -154.79267420126754, -153.3633238220272, -151.1769823593961, -150.52071361991585, -150.04865841374036, -147.2179444629798, -146.3815863379968, -148.42924058701334, -151.31521776248252, -153.05712615919353, -159.0181366666726, -168.42615356122766, -172.86891250543835, -160.02882246286566, -152.65834725885196, -149.78662596693707, -151.21074996968974, -155.33170909860357, -155.85490036822114, -150.75132404605958, -147.35334413001306, -146.25259009254424, -146.07305671822854, -145.3104684846153, -144.15013458965103, -143.53881162267027, -143.4974594864061, -143.4487592301008, -143.57333302894438, -143.75146076630892, -143.5167974846791, -143.60633323035796, -144.61419759191222, -146.02125022311427, -146.94284521390253, -147.58624345762092, -150.49060482898702, -160.01068623130496, -153.0718667169204, -150.5820319059295, -150.8719416099005, -154.45246363587307, -160.0422611512874, -151.8505258774379, -151.64072773621876, -151.30134355567174, -147.37448186156374, -145.57895477209965, -145.82303056685896, -147.31088517480111, -149.80657525645245, -153.298544571586, -156.0527940870806, -150.78741635240237, -145.59230953135224, -143.43713640951302, -143.23146624311303, -143.78261824049395, -145.4056357786411, -150.05923263520236, -152.51740519954868, -149.86023454359193, -151.41222085979197, -156.60157482486414, -154.61442946221874, -149.749810486032, -147.8802592679888, -149.13439875678097, -154.2940013366025, -160.2016880075399, -160.41706391146488, -155.81979329601444, -151.13067740925163, -150.8967063308886, -155.22311112488202, -151.36332854608963, -146.75014726826538, -144.62145432161253, -144.57499509559284, -147.99016790226196, -161.2684513303259, -154.77971508786388, -152.9335945175335, -155.03389006228673, -152.65271786410858, -149.41432544371287, -147.91531476668405, -146.51175597376655, -146.1667052465461, -148.39453902787886, -152.81241342354338, -158.38584364775403, -154.8680179009901, -150.7993947827226, -149.79765296404958, -150.42140625908982, -153.72867656881994, -156.3511366298644, -156.31285123769996, -173.88221564313196, -150.20765992324212, -144.73962350870588, -142.99450711166278, -144.16557902189783, -149.65008692319716, -164.23335597131032, -153.20992126481542, -152.98420618972852, -155.30562180599534, -155.77690099792284, -152.94377460465873, -148.0164478264011, -144.19969533781267, -142.40616540238273, -143.07446631472698, -146.54296222833054, -152.5325559944966, -153.66218521509944, -146.63014418469072, -142.83648318576473, -141.31655891522573, -141.7161451959318, -144.18885876977146, -147.77075664886777, -150.0161240727678, -152.30902938580473, -158.37402213196424, -154.76414843053448, -150.6881421448262, -150.81484828548528, -154.27259088416352, -150.31396763045296, -145.8541214895542, -144.64994221085328, -145.27959957710019, -147.2572507682597, -151.25380108325618, -158.97875491924205, -162.4732693320111, -156.09517901425986, -153.5448267320266, -150.95952741837306, -147.78366983663238, -148.50524223278848, -152.90582937302526, -150.05029549191232, -150.41493487650308, -147.94789198439315, -143.8365541564883, -144.5462054214396, -151.99953610115014, -161.8106482273226, -155.42134987438246, -157.37414110824423, -159.8082168631843, -165.7349703113813, -158.19808031017925, -155.30309813707572, -162.4917930069631, -145.55246796784772, -140.64561502429274, -139.2590943829006, -139.7941397128813, -141.81563966723144, -146.15378868834964, -157.60667296001762, -154.1382652329504, -151.59846957026394, -150.57091773435624, -148.31532873236736, -150.67582934439375, -158.44698122531568, -152.59609178160304, -147.87272747225072, -145.23752848099838, -145.14185599841213, -147.53519214924364, -151.2274137870829, -161.980566455869, -155.14836093214996, -149.8204982877691, -149.38489357259417, -150.88626611269015, -152.14134929430273, -150.3735103498207, -148.27520409212417, -148.5487486718063, -152.55477602518565, -162.40835748717555, -166.1883344331059, -172.84155047472694, -156.45755776134973, -146.92178261627342, -142.89609392698617, -141.50511129966958, -141.81095403614867, -144.45466449807043, -152.37880616703615, -157.97755862828072, -150.46301645184275, -149.90835305111344, -146.77611638366915, -143.84968844936785, -144.7733165830223, -149.99985530875549, -147.46517601435397, -144.79917751910864, -146.30685028813008, -147.45194183270837, -148.49202576680253, -155.0527382303689, -155.94678087029132, -151.08071652449263, -150.60105751940802, -152.08506309763843, -153.24643508673824, -153.06117308341683, -154.25082421271733, -162.0049754963412, -154.91638310125134, -148.97841483813468, -147.0588863891191, -146.8834580123894, -148.64786222687917, -151.60264959731035, -149.5574672028649, -146.21534572296028, -145.5803087986676, -148.17579419428267, -153.0536880310635, -154.6713532184287, -154.54195134672216, -156.8070886861977, -162.1803213511368, -150.50431536676848, -147.44216033626074, -146.89465984123007, -144.78731284585908, -143.36257314413098, -143.852954405759, -145.17423180865956, -145.51754672753395, -144.94978999264075, -145.40906971538408, -145.82568948094877, -144.7635204487679, -145.6543306283464, -149.64404115451546, -154.18404466630616, -153.7153050021356, -150.28803563525128, -149.80062504826103, -152.4522219338782, -154.55580920182126, -149.75657921846417, -148.34638945510082, -149.64610738566944, -147.63298811987585, -144.3557747785122, -143.53336540906378, -145.6524739311589, -150.3916684193967, -155.5317606182494, -164.0123587531408, -158.3967343274771, -152.60906881903168, -152.90466072930894, -153.294328149752, -150.26100449386172, -148.1607688856398, -146.80970218658877, -145.5094910739165, -145.40556354344758, -148.8174987608062, -154.64759367550235, -146.56881007004722, -144.4830826662199, -145.62858870081675, -145.05271579819026, -144.18981403682918, -146.49016871322567, -155.34600062193272, -156.72709593122119, -148.24441524787554, -145.993173787172, -146.52047349999737, -147.4013832100769, -146.66319390820806, -146.32253642489619, -148.16530184586654, -153.32874433341456, -162.93081730836118, -152.48668712776077, -151.80081908936626, -159.58750217727322, -160.5548420820219, -166.46835313876667, -162.54861487599086, -157.61711233558634, -148.70573699907743, -146.0419329854272, -148.00076663462946, -153.6538710882508, -158.99853261628607, -158.9262277486053, -158.46875938308222, -159.2143691068846, -154.35927614154554, -148.4732722465141, -145.18738455583804, -144.428314491718, -146.3995525653781, -148.34073711787704, -146.4159210793544, -145.14993596055987, -144.752138461966, -144.96336818721704, -146.7059108653912, -151.74645536177516, -158.21109520408208, -153.62181795594876, -154.44051306957792, -157.5001825800422, -159.09481649918362, -153.54302691237547, -153.14996966034647, -157.0085182635812, -150.3764148587289, -148.3910993892475, -151.80003385503267, -158.36646296565476, -156.74818533694548, -155.090254690208, -153.00882053734196, -152.54343687068098, -155.86910355641675, -155.1052300704723, -152.35440644809432, -155.81257818007387, -164.38712971143735, -150.26673467741165, -147.2938449354303, -147.56931725001448, -147.44857065251796, -146.29956143625967, -145.12954035647735, -145.198106234288, -147.09108858272094, -148.93018066148713, -148.17966774060625, -146.9689743174684, -147.55306661408252, -150.18794872644688, -153.25985023462698, -153.94151859881242, -153.48013682416698, -152.76281649048545, -150.70250239375602, -148.5564071457321, -148.01457715305563, -149.15123137415867, -150.66289995150478, -150.04453734316075, -146.82792740181372, -145.20530646699683, -145.66113375816917, -147.17235794114424, -150.0730013073184, -155.55541537150427, -154.43204682779236]}, ...(2 in all)]
  out "Waveform Graph":waveform(dbl)[](graph)=[{"t0"=timestamp(3785947881.0962696 s since 1904-01-01), "dt"=1.9531249997269942e-05, "Y"=array[5120 elements], "attributes"=variant("NI_ChannelName"=variant(string "PXI1Slot4/ai1"), "NI_UnitDescription"=variant(string "Volts"))}, {"t0"=timestamp(3785947881.0962696 s since 1904-01-01), "dt"=1.9531249997269942e-05, "Y"=array[5120 elements], "attributes"=variant("NI_ChannelName"=variant(string "PXI1Slot4/ai0"), "NI_UnitDescription"=variant(string "Volts"))}]
  out "Measurement Context out":refnum<class "MeasurementContext.lvclass">
  in  "Measurement Context":refnum<class "MeasurementContext.lvclass">=refnum
  out "Measurement Results":T1={"channel name"="", "measured frequency (Hz)"=999.9999805150366, "crosstalk (dB)"=-96.02835709393884, "output power (W)"=0.0, "wfm - dt"=1.9531249997269942e-05, "wfm_victim - data"=array[5120 elements], "wfm_interferrer - data"=array[5120 elements], "fft - f0"=0.0, "fft - df"=10.00000000139779, "fft_victim - data"=array[2560 elements], "fft_interferrer - data"=array[2560 elements]}
  in  "Measurement Configuration":T2={"digital channel list"="7821\\PCMo 8", "frame clock rate"=48000.0, "number of channels"=2, "channel length"=32, "bit depth"=24, "data justification"=enum."Left Justified", "endianness"=enum."MSB First", "bit clock edge sync"=enum."Falling", "frame sync edge for channel 0"=enum."Falling", "channel 0 offset"=1, "master clock channel list"="7821\\PCMo 0", "master clock rate"=12288000.0, "digital audio interferrer channel"=0, "logic level"=enum."3.3 V", "signal frequency"=1000.0, "output mode"=enum."Level", "output level (dB)"=-1.0, "output power (W)"=1.0, "output range (pk-pk)"=14.4, "load impedance"=4.0, "signal phase"=0.0, "acq sampling rate"=51200.0, "min measurement cycles"=0, "min measurement time (s)"=5.0, "min settling cycles"=0, "min settling time (s)"=0.0, "acq channel - victim"="PXI1Slot4/ai1", "acq channel - interferrer"="PXI1Slot4/ai0", "lowpass filter"=enum."No filter", "highpass filter"=enum."DC"} {"min measurement cycles" format="%.3f"; "load impedance" format="%.2f"; "channel 0 offset" format="%#_6p"; "output range (pk-pk)" format="%0.2f"; "acq sampling rate" format="%0.2f"; "output level (dB)" format="%0.2f"; "frame clock rate" format="%#_6pHz"}
  out "error out":errorcluster
  in  "error in":errorcluster
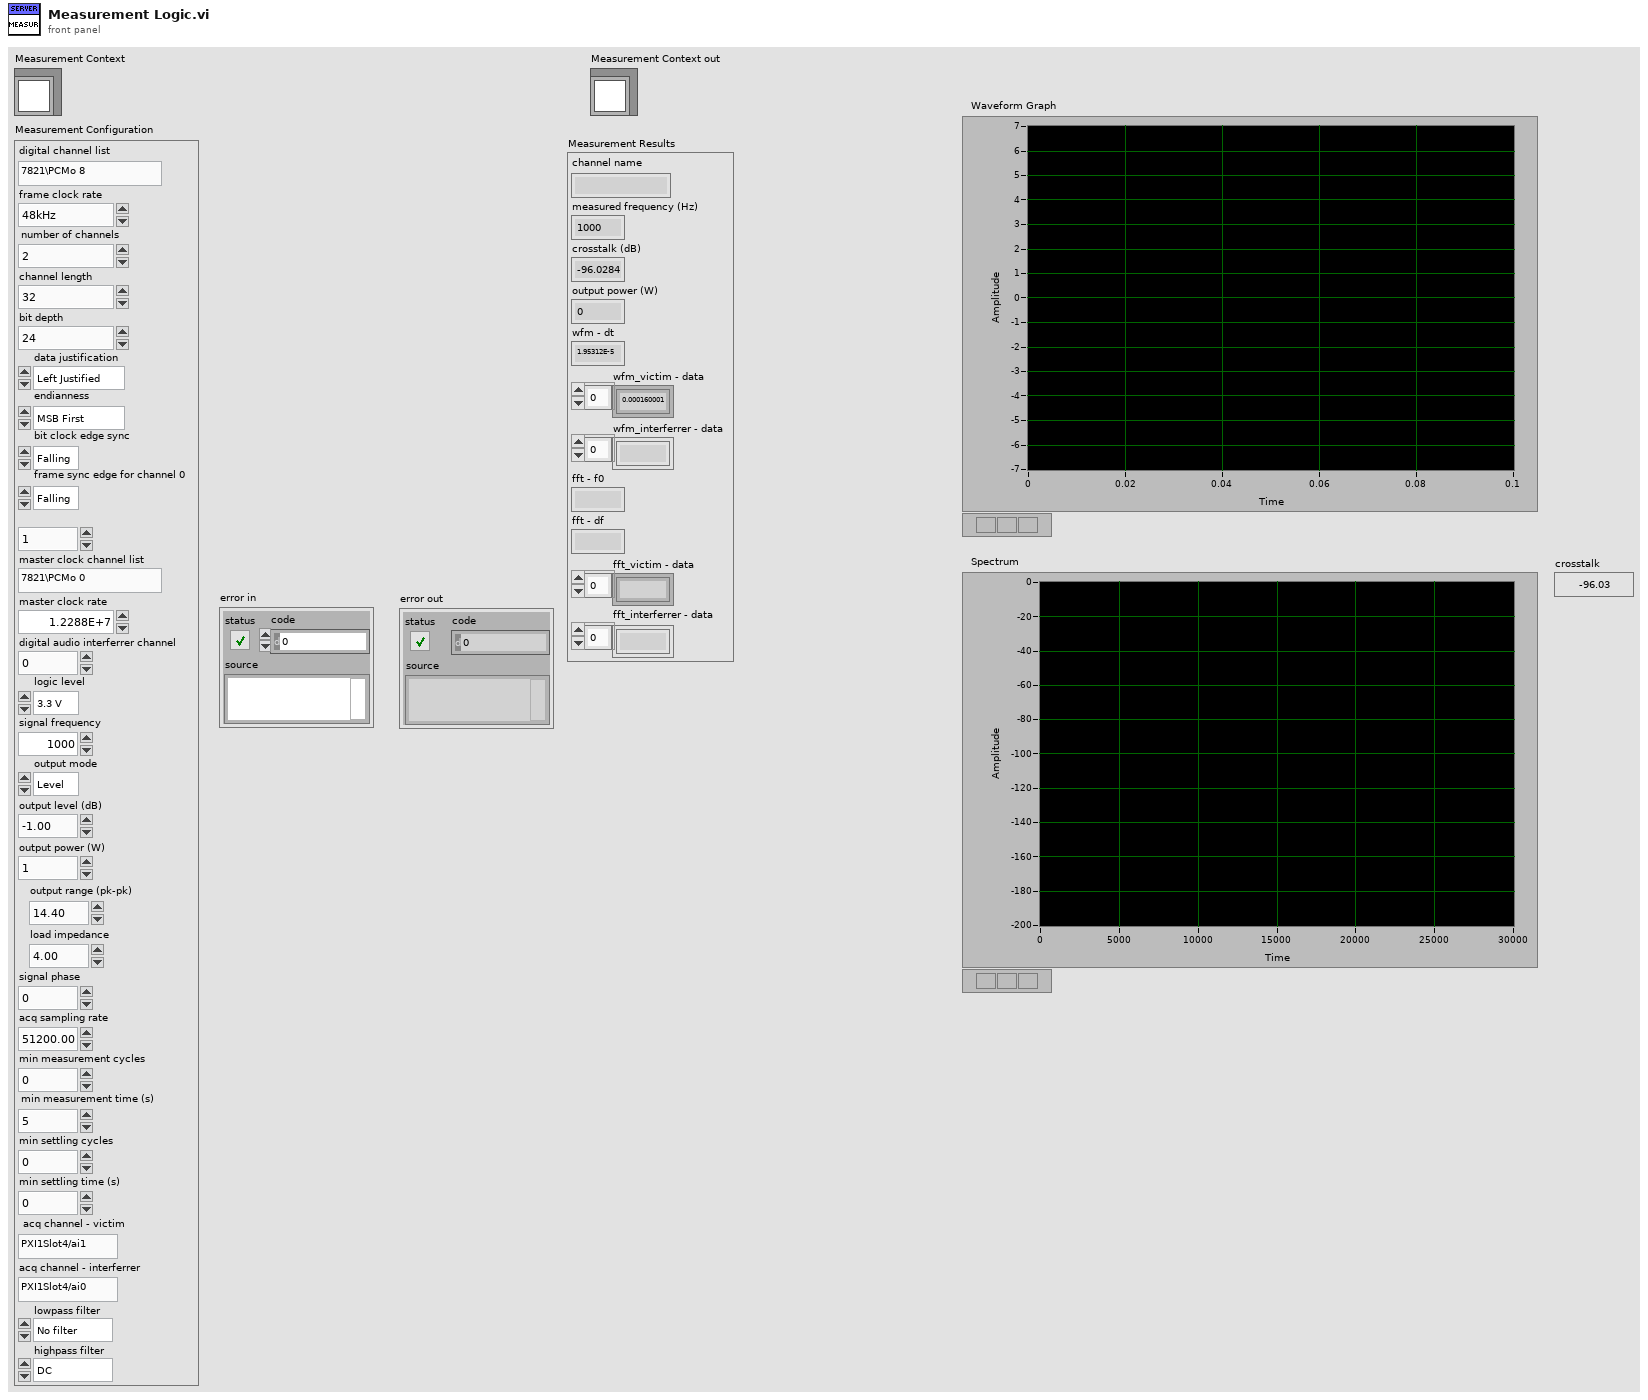
[diagram p1: front panel]
types:
  T1 = typedef "Crosstalk_Class D Amplifier.lvlib/Measurement Results.ctl" = cluster{"channel name":string, "measured frequency (Hz)":dbl, "crosstalk (dB)":dbl, "output power (W)":dbl, "wfm - dt":dbl, "wfm_victim - data":dbl[], "wfm_interferrer - data":dbl[], "fft - f0":dbl, "fft - df":dbl, "fft_victim - data":dbl[], "fft_interferrer - data":dbl[]}
  T2 = typedef "Crosstalk_Class D Amplifier.lvlib/Measurement Configuration.ctl" = cluster{"digital channel list":string, "frame clock rate":dbl, "number of channels":u32, "channel length":u32, "bit depth":u32, "data justification":T3, "endianness":T4, "bit clock edge sync":T5, "frame sync edge for channel 0":T5, "channel 0 offset":u32, "master clock channel list":string, "master clock rate":dbl, "digital audio interferrer channel":i32, "logic level":T6, "signal frequency":dbl, "output mode":T7, "output level (dB)":dbl, "output power (W)":dbl, "output range (pk-pk)":dbl, "load impedance":dbl, "signal phase":dbl, "acq sampling rate":dbl, "min measurement cycles":u32, "min measurement time (s)":dbl, "min settling cycles":u32, "min settling time (s)":dbl, "acq channel - victim":string, "acq channel - interferrer":string, "lowpass filter":T8, "highpass filter":T9}
  T3 = typedef "data justification.ctl" = enum32{"Left Justified", "Right Justified"}
  T4 = typedef "endianness.ctl" = enum32{"MSB First", "LSB First"}
  T5 = typedef "digital edge.ctl" = enum32{"Rising", "Falling"}
  T6 = typedef "logic level.ctl" = enum32{"3.3 V", "1.8 V", "1.2 V"}
  T7 = typedef "output mode.ctl" = enum32{"Level", "Power"}
  T8 = typedef "lowpass filter.ctl" = enum32{"No filter", "AES17 20kHz", "AES17 40kHz"}
  T9 = typedef "highpass filter.ctl" = enum32{"DC", "AC"}
  T10 = typedef "weighting filter.ctl" = enum32{"Linear", "A-weighting", "B-weighting", "C-weighting"}
  T11 = typedef "audio filter settings.ctl" = cluster{"weighting filter":T10, "highpass filter":T9, "lowpass filter ":T8}
  T12 = cluster{"linear/dB":enum16{"no change", "linear", "dB"}, "dB reference (0: no change)":dbl, "power/magnitude":enum16{"no change", "power", "magnitude"}, "view":enum16{"no change", "rms", "peak", "peak-peak"}}
  T13 = typedef "PDM Shared.lvlib/PCM Data Format Configuration.ctl" = cluster{"Frame Sync Edge for Channel 0":T14, "Channel Count Per Frame":u8, "Channel Length":u16, "Bit Depth":u8, "Channel 0 Offset":u16, "Endianness":T15, "Data Justification":T16}
  T14 = typedef "PDM Shared.lvlib/Digital Edge.ctl" = enum8{"Rising", "Falling"}
  T15 = typedef "PDM Shared.lvlib/PCM Bit Endianness.ctl" = enum16{"MSB First", "LSB First"}
  T16 = typedef "PDM Shared.lvlib/PCM Data Justification.ctl" = enum16{"Left Justified", "Right Justified"}
  T17 = typedef "PDM Shared.lvlib/PCM Frame Sync Control.ctl" = cluster{"Frame Length":u16, "Frame Sync Pulse Width":u16, "Bit Clock Edge  Sync":T14}
  T18 = typedef "PDM Shared.lvlib/clock mode.ctl" = enum16{"divided clock", "DDS"}
  T19 = typedef "PDM Acquisition Class Library.lvlib/PCM Output Task.lvclass/PCM Output Task DVR.ctl" = refnum<data-value>
  T20 = typedef "PDM Acquisition Class Library.lvlib/I2S Output Task.lvclass/SignalProperties.ctl" = cluster{"cyclic signal":dbl[], "channel parameters":T21[]}
  T21 = typedef "PDM Acquisition Class Library.lvlib/I2S Output Channel.lvclass/GenerationChannelProperties.ctl" = cluster{"cyclic period":dbl, "cyclic phase offset":dbl, "gain":dbl}
  T22 = typedef "svc_Spectrum Info.ctl" = cluster{"channel name":string, "description":string, "x-axis units":T23, "spectral info":cluster{"spectrum type":T24, "linear/dB":enum16{"linear", "dB"}, "window":u16, "window size":i32, "FFT size":i32}, "engineering units":T25, "custom label":string, "dB reference [EU]":dbl, "peak units":enum16{"rms", "peak", "peak-peak"}, "weighting filter":T26, "spectral density?":bool, "unit label":string, "spectrum skewed?":bool, "complimentary spectrum units":T27}
  T23 = typedef "svc_X-Axis Units.ctl" = u16
  T24 = typedef "svc_Spectrum Type.ctl" = enum16{"FFT Spectrum [complex]", "Amplitude [Magnitude]", "Power [Magnitude^2]", "Cross Spectrum [complex]", "Frequency Response [Complex]"}
  T25 = typedef "svc_Engineering Units Text Ring.ctl" = u16
  T26 = typedef "svc_Weighting Filter Text Ring.ctl" = u16
  T27 = typedef "svc_Complimentary Spectrum Units.ctl" = enum16{"none", "radians", "degrees", "cycles", "imaginary"}
  T28 = cluster{"complex spectrum response":cluster{"f0":dbl, "df":dbl, "complex spectrum":cdb[]}, "spectrum info":T22}
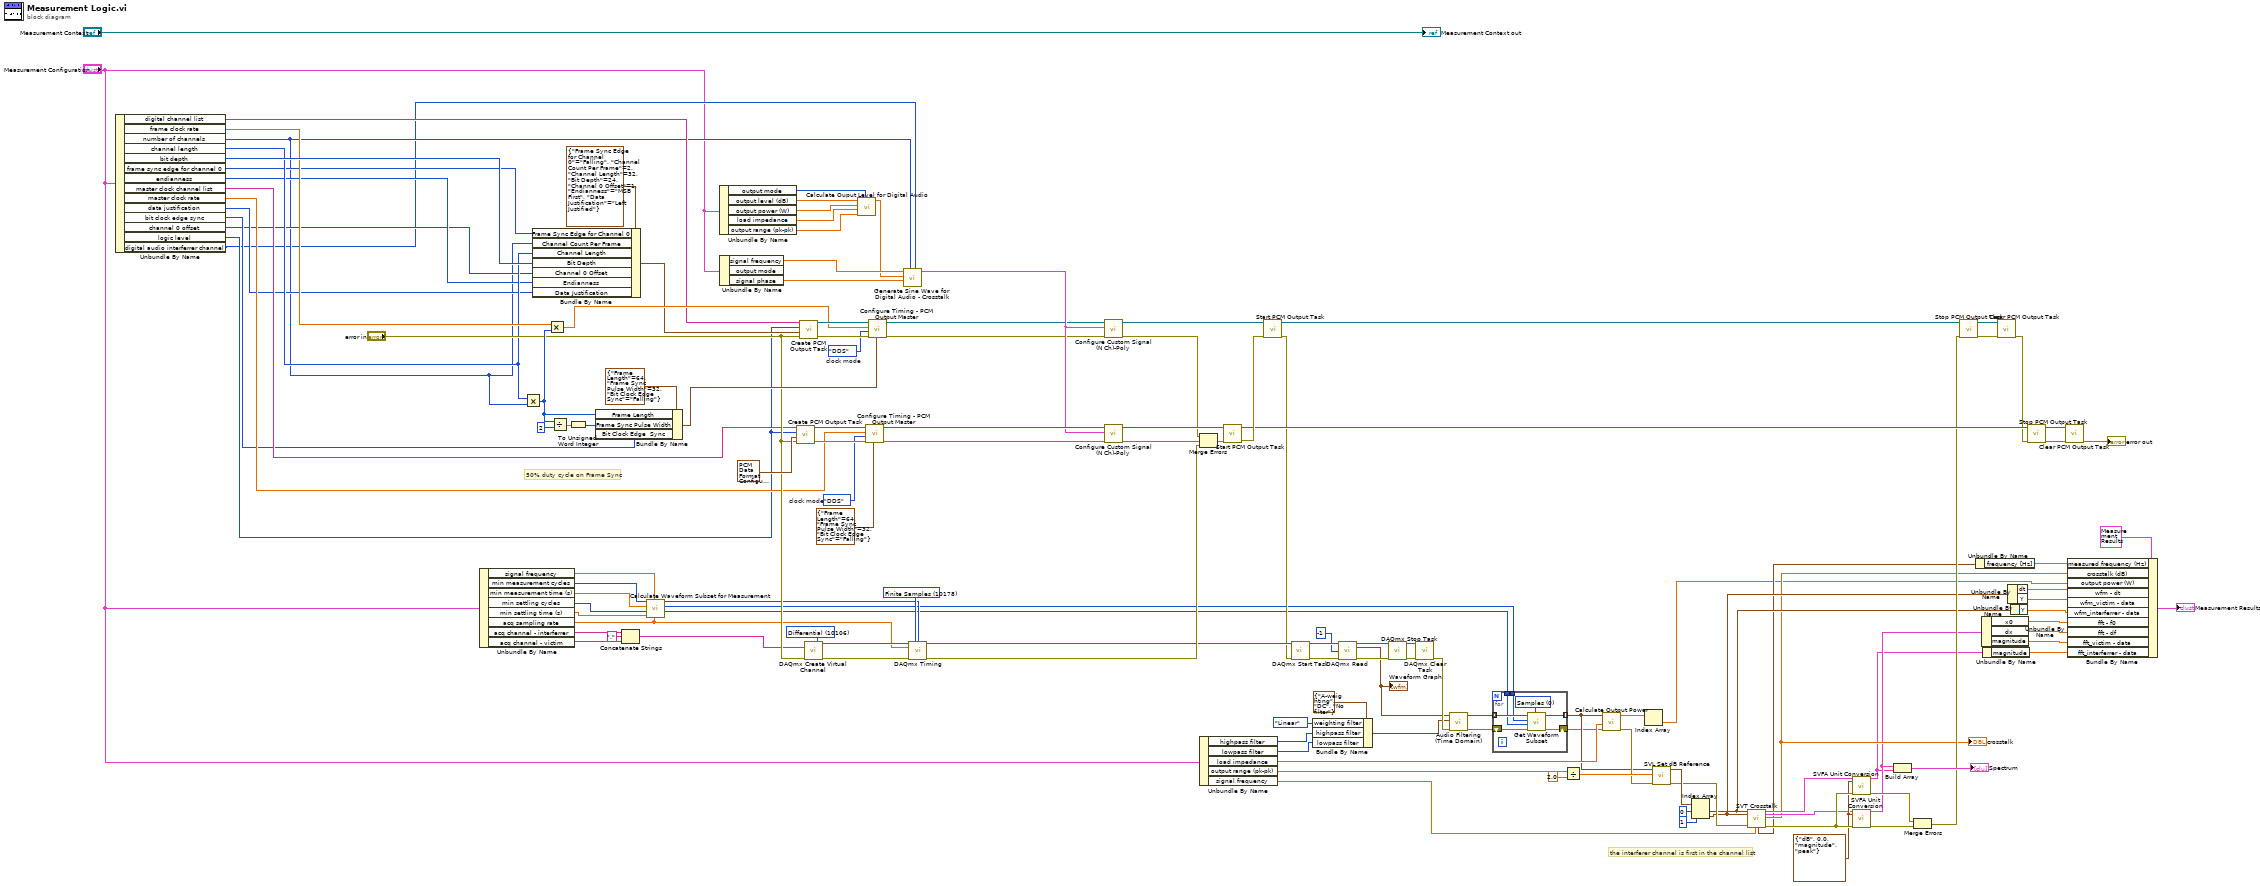
[diagram p0: block diagram]
diagram:
  w67 = T12 {"linear/dB"=enum."dB", "dB reference (0: no change)"=0.0, "power/magnitude"=enum."magnitude", "view"=enum."peak"} ("desired scaling")
  w79 = 10106 items=["Default"=-1, "RSE"=10083, "NRSE"=10078, "Differential"=10106, "Pseudodifferential"=12529] ("input terminal configuration")
  w89 = 10178 items=["Finite Samples"=10178, "Continuous Samples"=10123, "Hardware Timed Single Point"=12522] ("sample mode")
  w126 = clock_mode."DDS"  # clock mode
  w129 = clock_mode."DDS"  # clock mode
  # "the interferer channel is first in the channel list"
  # "50% duty cycle on Frame Sync"
  n1 = Unbundle By Name("Measurement Configuration") -> ("digital channel list"=w85:string, "frame clock rate"=w83:dbl, "number of channels"=w35:u32, "channel length"=w82:u32, "bit depth"=w84:u32, "frame sync edge for channel 0"=w76:T5, "endianness"=w75:T4, "master clock channel list"=w81:string, "master clock rate"=w80:dbl, "data justification"=w77:T3, "bit clock edge sync"=w74:T5, "channel 0 offset"=w73:u32, "logic level"=w72:T6, "digital audio interferrer channel"=w34:i32)
  n2 = Unbundle By Name("Measurement Configuration") -> ("signal frequency"=w13:dbl, "min measurement cycles"=w12:u32, "min measurement time (s)"=w11:dbl, "min settling cycles"=w10:u32, "min settling time (s)"=w9:dbl, "acq sampling rate"=w8:dbl, "acq channel - interferrer"=w44:string, "acq channel - victim"=w43:string)
  n3 = Multiply(x=w82, y=w35) -> (x*y=w112:u32)
  n4 = Bundle By Name(cluster=T13 {"Frame Sync Edge for Channel 0"=enum."Falling", "Channel Count Per Frame"=2, "Channel Length"=32, "Bit Depth"=24, "Channel 0 Offset"=1, "Endianness"=enum."MSB First", "Data Justification"=enum."Left Justified"} ("PCM Data Configuration"), "Frame Sync Edge for Channel 0"=w76, "Channel Count Per Frame"=w35, "Channel Length"=w82, "Bit Depth"=w84, "Channel 0 Offset"=w73, "Endianness"=w75, "Data Justification"=w77) -> (w109:T13)
  n5 = Multiply(x=w83, y=w112) -> (x*y=w111:dbl)
  n6 = Divide(x=w112, y=u16 2) -> (x/y=w114:dbl)
  n7 = To Unsigned Word Integer(number=w114) -> (unsigned 16bit integer=w113:u16)
  n8 = Bundle By Name(cluster=T17 {"Frame Length"=64, "Frame Sync Pulse Width"=32, "Bit Clock Edge  Sync"=enum."Falling"} ("Frame Sync Clock Control"), "Frame Length"=w112, "Frame Sync Pulse Width"=w113, "Bit Clock Edge  Sync"=w74) -> (w116:T17)
  n9 = Concatenate Strings(w44, "," ("string"), w43) -> (w41:string)
  n10 = call "Calculate Waveform Subset for Measurement.vi"("sampling rate"=w8, "signal frequency"=w13, "minimum settling duration"=w9, "minimum settling cycles"=w10, "minimum measurement duration"=w11, "minimum measurement cycles"=w12) -> ("duration (samples)"=w6:u32, "start (samples)"=w7:u32, "total acquisition (samples)"=w14:u32)  [unwired: 3 in]
  n11 = Unbundle By Name("Measurement Configuration") -> ("output mode"=w31:T7, "output level (dB)"=w30:dbl, "output power (W)"=w29:dbl, "load impedance"=w28:dbl, "output range (pk-pk)"=w27:dbl)
  n12 = Unbundle By Name("Measurement Configuration") -> ("signal frequency"=w86:dbl, "signal phase"=w87:dbl)  [unwired: 1 out]
  n13 = call <vilib>:"Create PCM Output Task.vi"("error in"="error in", "PCM data configuration"=T13 {"Frame Sync Edge for Channel 0"=enum."Falling", "Channel Count Per Frame"=2, "Channel Length"=32, "Bit Depth"=24, "Channel 0 Offset"=1, "Endianness"=enum."MSB First", "Data Justification"=enum."Left Justified"} ("PCM Data Configuration 2"), "logic level"=w72, "channel list"=w81) -> ("error out"=w127:errorcluster, "PCM output task out"=w128:T19)  [unwired: 6 in]
  n14 = call <vilib>:"Create PCM Output Task.vi"("error in"="error in", "PCM data configuration"=w109, "logic level"=w72, "channel list"=w85) -> ("error out"=w130:errorcluster, "PCM output task out"=w131:T19)  [unwired: 6 in]
  n15 = call-poly <vilib>:"DAQmx Create Virtual Channel.vi"("input terminal configuration"=w79, "physical channels"=w41, "error in"="error in") -> ("task out"=w99:refnum<k21>, "error out"=w100:errorcluster)  [unwired: 11 in]
  n16 = call "Calculate Ouput Level for Digital Audio.vi"("output mode"=w31, "output range (pk-pk)"=w27, "load impedance"=w28, "output power (W)"=w29, "output level (dB)"=w30) -> ("gain"=w26:dbl)  [unwired: 5 in, 1 out]
  n17 = call <vilib>:"Configure Timing - PCM Output Master.vi"("Frame Sync Clock Control"=T17 {"Frame Length"=64, "Frame Sync Pulse Width"=32, "Bit Clock Edge  Sync"=enum."Falling"} ("Frame Sync Clock Control 2"), "error in"=w127, "clock mode"=w126, "Bit Clock rate"=w80, "PCM output task in"=w128) -> ("error out"=w108:errorcluster, "PCM output task out"=w107:T19)  [unwired: 4 in, 1 out]
  n18 = call <vilib>:"Configure Timing - PCM Output Master.vi"("Frame Sync Clock Control"=w116, "error in"=w130, "clock mode"=w129, "Bit Clock rate"=w111, "PCM output task in"=w131) -> ("error out"=w32:errorcluster, "PCM output task out"=w33:T19)  [unwired: 4 in, 1 out]
  n19 = call "Generate Sine Wave for Digital Audio - Crosstalk.vi"("interferrer channel"=w34, "number of channels"=w35, "phase"=w87, "gain"=w26, "frequency"=w86) -> ("Signal Properties"=w36:T20)  [unwired: 6 in]
  n20 = call-poly <vilib>:"DAQmx Timing.vi"("task/channels in"=w99, "sample mode"=w89, "samples per channel"=w14, "rate"=w8, "error in"=w100) -> ("task out"=w90:refnum<k21>, "error out"=w91:errorcluster)  [unwired: 9 in]
  n21 = call-poly <vilib>:"Configure Custom Signal (N Ch)-Poly.vi"("error in"=w32, "signal parameters"=w36, "PCM output task in"=w33) -> ("error out"=w104:errorcluster, "PCM output task out"=w105:T19)  [unwired: 7 in]
  n22 = call-poly <vilib>:"Configure Custom Signal (N Ch)-Poly.vi"("error in"=w108, "signal parameters"=w36, "PCM output task in"=w107) -> ("error out"=w103:errorcluster, "PCM output task out"=w106:T19)  [unwired: 7 in]
  n23 = Merge Errors(w104, w103, w91) -> (w122:errorcluster)
  n24 = Unbundle By Name("Measurement Configuration") -> ("highpass filter"=w3:T9, "lowpass filter"=w2:T8, "load impedance"=w22:dbl, "output range (pk-pk)"=w46:dbl, "signal frequency"=w48:dbl)
  n25 = call <vilib>:"Start PCM Output Task.vi"("error in"=w122, "PCM output task in"=w106) -> ("error out"=w123:errorcluster, "PCM output task out"=w119:T19)  [unwired: 8 in]
  n26 = call <vilib>:"Start PCM Output Task.vi"("error in"=w123, "PCM output task in"=w105) -> ("error out"=w78:errorcluster, "PCM output task out"=w102:T19)  [unwired: 8 in]
  n27 = call <vilib>:"DAQmx Start Task.vi"("task/channels in"=w90, "error in"=w78) -> ("task out"=w94:refnum<k21>, "error out"=w97:errorcluster)  [unwired: 12 in]
  n28 = Bundle By Name(cluster=T11 {"weighting filter"=enum."A-weighting", "highpass filter"=enum."DC", "lowpass filter "=enum."No filter"} ("filter settings"), "weighting filter"=weighting_filter."Linear", "highpass filter"=w3, "lowpass filter"=w2) -> (w4:T11)
  n29 = call-poly <vilib>:"DAQmx Read.vi"("task/channels in"=w94, "number of samples per channel"=-1, "error in"=w97) -> ("task out"=w93:refnum<k21>, "data"=w17:waveform(dbl)[], "error out"=w96:errorcluster)  [unwired: 10 in]
  "Waveform Graph" <- w17
  n30 = call <vilib>:"DAQmx Stop Task.vi"("task/channels in"=w93, "error in"=w96) -> ("task out"=w98:refnum<k21>, "error out"=w95:errorcluster)  [unwired: 12 in]
  n31 = call <vilib>:"DAQmx Clear Task.vi"("task in"=w98, "error in"=w95) -> ("error out"=w18:errorcluster)  [unwired: 13 in]
  n32 = call "Audio Filtering (Time Domain).vi"("waveforms"=w17, "filter settings"=w4, "error in"=w18) -> ("time domain"=w19:waveform(dbl)[], "error out"=w20:errorcluster)  [unwired: 6 in]
  n33 = for {
    tunnel: w19 -> [w142] mode=indexing
    tunnel: [w141] -> w16 mode=indexing
    shift-right: [w138] -> w15
    shift-left: w20 -> [w139]
    tunnel: w7 -> [w137]
    tunnel: w6 -> [w136]
    w140 = u16 0 items=["Samples", "Relative Time"] ("start/duration format")
    n34 = call-poly <vilib>:"Get Waveform Subset.vi"("start/duration format"=w140, "error in (no error)"=w139, "duration"=w136, "start samples/time"=w137, "waveform in"=w142) -> ("error out"=w138:errorcluster, "waveform out"=w141:waveform(dbl))  [unwired: 1 in, 2 out]
  }
  n35 = Divide(x=w46, y=2.0) -> (x/y=w47:dbl)
  n36 = call "Calculate Output Power.vi"("error in (no error)"=w15, "load impedance"=w22, "waveforms"=w16) -> ("error out"=w24:errorcluster, "output power"=w23:dbl[])  [unwired: 7 in]
  n37 = Index Array(array=w23) -> (element=w21:dbl)  [unwired: 1 in]
  n38 = call-poly <vilib>:"SVL Set dB Reference.vi"("error in (no error)"=w24, "dB reference [EU]"=w47, "scaled signals in [EU]"=w16) -> ("error out"=w64:errorcluster, "scaled signals out [EU]"=w65:waveform(dbl)[])  [unwired: 7 in]
  n39 = Index Array(array=w65, index #1=0 ("index"), index #2=1 ("index")) -> (element #1=w62:waveform(dbl), element #2=w60:waveform(dbl))
  n40 = call-poly <vilib>:"SVT Crosstalk.vi"("stimulus signal X [EUx]"=w62, "idle-channel response signal Y [EUy]"=w60, "error in (no error)"=w64, "expected fundamental frequency [Hz]"=w48) -> ("detected tone idle-channel response"=w50:cluster{"frequency [Hz]":dbl, "amplitude":dbl}, "complex spectrum\nstimulus X"=w71:T28, "complex spectrum\nidle-channel response Y"=w57:T28, "crosstalk"=w51:dbl, "error out"=w70:errorcluster)  [unwired: 8 in, 3 out]
  "crosstalk" <- w51
  n41 = call-poly <vilib>:"SVFA Unit Conversion.vi"("complex spectrum"=w71, "desired scaling"=w67, "error in (no error)"=w70) -> ("converted spectrum"=w37:cluster{"x0":dbl, "dx":dbl, "magnitude":dbl[]}, "error out"=w68:errorcluster)  [unwired: 11 in, 4 out]
  n42 = call-poly <vilib>:"SVFA Unit Conversion.vi"("complex spectrum"=w57, "desired scaling"=w67, "error in (no error)"=w70) -> ("converted spectrum"=w38:cluster{"x0":dbl, "dx":dbl, "magnitude":dbl[]}, "error out"=w69:errorcluster)  [unwired: 11 in, 4 out]
  n43 = Build Array(w38, w37) -> (→"Spectrum":cluster{"x0":dbl, "dx":dbl, "magnitude":dbl[]}[])
  n44 = Merge Errors(w68, w69) -> (w63:errorcluster)
  n45 = call <vilib>:"Stop PCM Output Task.vi"("error in"=w63, "PCM output task In"=w102) -> ("error out"=w133:errorcluster, "PCM output task out"=w132:T19)  [unwired: 8 in]
  n46 = Unbundle By Name(w50) -> ("frequency [Hz]"=w49:dbl)
  n47 = Unbundle By Name(w38) -> ("x0"=w56:dbl, "dx"=w55:dbl, "magnitude"=w54:dbl[])
  n48 = Unbundle By Name(w37) -> ("magnitude"=w53:dbl[])
  n49 = call <vilib>:"Clear PCM Output Task.vi"("error in"=w133, "PCM output task in"=w132) -> ("error out"=w118:errorcluster)  [unwired: 9 in]
  n50 = Unbundle By Name(w60) -> ("dt"=w58:dbl, "Y"=w59:dbl[])
  n51 = Unbundle By Name(w62) -> ("Y"=w61:dbl[])
  n52 = call <vilib>:"Stop PCM Output Task.vi"("error in"=w118, "PCM output task In"=w119) -> ("error out"=w121:errorcluster, "PCM output task out"=w120:T19)  [unwired: 8 in]
  n53 = call <vilib>:"Clear PCM Output Task.vi"("error in"=w121, "PCM output task in"=w120) -> ("error out"=→"error out":errorcluster)  [unwired: 9 in]
  n54 = Bundle By Name(cluster=T1 {"channel name"="", "measured frequency (Hz)"=0.0, "crosstalk (dB)"=0.0, "output power (W)"=0.0, "wfm - dt"=0.0, "wfm_victim - data"=[], "wfm_interferrer - data"=[], "fft - f0"=0.0, "fft - df"=0.0, "fft_victim - data"=[], "fft_interferrer - data"=[]} ("Measurement Results"), "measured frequency (Hz)"=w49, "crosstalk (dB)"=w51, "output power (W)"=w21, "wfm - dt"=w58, "wfm_victim - data"=w59, "wfm_interferrer - data"=w61, "fft - f0"=w56, "fft - df"=w55, "fft_victim - data"=w54, "fft_interferrer - data"=w53) -> (→"Measurement Results":T1)
  "Measurement Context out" <- "Measurement Context"
